vi "Create Sessions.vi"   [LabVIEW 2020, in "MeasurementLink niScope.lvlib"]
doc: "Create the NI-SCOPE driver session(s) from a reservation."
uses:
  MeasurementLink niScope.lvlib
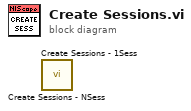
[diagram p0: block diagram]
diagram:
  n1 = call "Create Sessions - NSess.vi"() -> ()  [unwired: 8 in, 4 out]
  n2 = call "Create Sessions - 1Sess.vi"() -> ()  [unwired: 8 in, 4 out]
